vi "Create Message Group.vi"(8 "error in (no error)":errorcluster, 10 "Message Group Name":string, 11 "Instrument Addon Refnum In":T1 format="%.0x") -> (0 "error out":errorcluster, 2 "Message Group Refnum":T1 format="%.0x", 3 "Instrument Addon Refnum Out":T2=18446744073709551615 format="%.0x")   [LabVIEW 2018, in "Instrument Addon Scripting API.lvlib"]
uses:
  Instrument Addon Scripting API.lvlib
  Types/Instrument Addon Refnum In.ctl
  <vilib>/NI Veristand/Custom Device API/Custom Device Item Ref.ctl
  Addon/Addon Shared/SubVIs/Constants.vi
  <vilib>/NI VeriStand/Custom Device API/Custom Device API.lvlib
  Addon/Addon Shared/Instrument Addon Shared.lvlib
  <vilib>/NI VeriStand/Custom Device Tools/Custom Device Utility Library/Custom Device Utility Library.lvlib
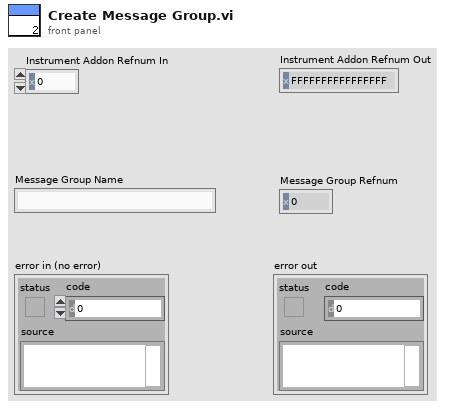
[diagram p1: front panel]
types:
  T1 = typedef "Instrument Addon Refnum In.ctl" = u64
  T2 = typedef "Custom Device API.lvlib/Custom Device Item Ref.ctl" = u64
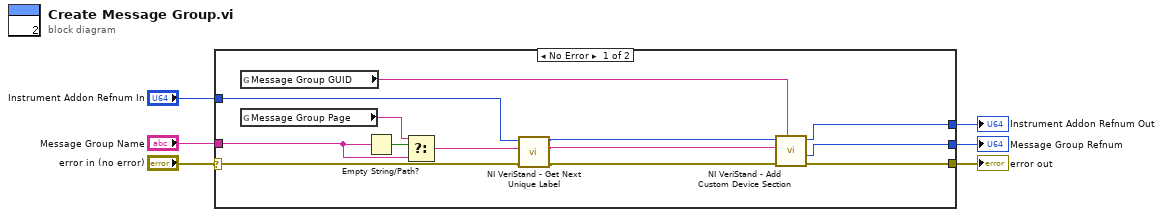
[diagram p0: block diagram]
diagram:
  n1 = case shown="No Error" "error in (no error)" {
    selector: "error in (no error)" -> [w9 w21]
    tunnel: "Message Group Name" -> [w16 _]
    tunnel: "Instrument Addon Refnum In" -> [w12 w20]
    tunnel: [w15 w21] -> w4
    tunnel: [w14 _] -> w1
    tunnel: [w13 w20] -> w2
    frame No Error {
      n2 = global read "Constants.vi" "Message Group GUID"() -> (w19:string)
      n3 = global read "Constants.vi" "Message Group Page"() -> (w17:string)
      n4 = Empty String/Path?(string/path=w16) -> (empty?=w18:bool)
      n5 = Select(t=w17, s=w18, f=w16) -> (s? t:f=w10:string)
      n6 = call <vilib>:"NI VeriStand - Get Next Unique Label.vi"("error in (no error)"=w9, "Label"=w10, "Parent Ref in"=w12) -> ("error out"=w8:errorcluster, "Label out"=w7:string, "Parent Ref dup"=w11:T2)  [unwired: 5 in, 1 out]
      n7 = call <vilib>:"NI VeriStand - Add Custom Device Section.vi"("GUID (Default Section)"=w19, "error in (no error)"=w8, "Section Name"=w7, "Parent Ref in"=w11) -> ("error out"=w15:errorcluster, "Section Ptr"=w14:T2, "Parent Ref out"=w13:T2)  [unwired: 4 in, 1 out]
    }
    frame Error {
    }
  }
  "error out" <- w4
  "Instrument Addon Refnum Out" <- w2
  "Message Group Refnum" <- w1
